vi "SQL_Table_Test_Time_Judge.vi"() -> ()   [LabVIEW 2014]
panel:
  in  "起始时间":timestamp=timestamp(3517116513.32069 s since 1904-01-01) format="%<%H:%M:%S\n%x>T"
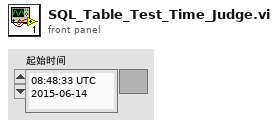
[diagram p1: front panel]
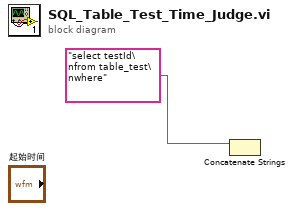
[diagram p0: block diagram]
diagram:
  n1 = Concatenate Strings("select testId\nfrom table_test\nwhere") -> ()  [unwired: 1 in, 1 out]
